vi "Mindsensors NXTMMX Config.vi"(10 "Node Data":T2, 11 "NXT":T3) -> ()   [LabVIEW 2010]
uses:
  <vilib>/NXT/Subs/LVHSConnector.ctl
  Datatypes/Node.ctl
  UI Controls/PlugInControls/Pluginbackground.ctl
  <vilib>/NXT/Block Support/nxt.ctl
  <vilib>/Utility/miscctls.llb/LVPointTypeDef.ctl
  <vilib>/NXT/Block Support/HWPage.SensorMode.ctl
  <vilib>/NXT/Block Support/HWPage.SensorType.ctl
  ConvertNodeAddrSensor.vi
panel:
  out "error out":errorcluster
  out "NXTObject dup":T1 {"nxtIterHandle" format="%08x"; "modIterHandle" format="%08x"; "moduleHandle" format="%08x"; "fileIterHandle" format="%08x"; "fileHandle" format="%08x"; "nxtHandle" format="%08x"}
  in  "Motor Control":string
  in  "Motor 2 Power":i32 min=-100 max=100 step=1
  in  "Motor 1 Power":i32 min=-100 max=100 step=1
  in  "Device Addr":u8=176 format="%x"
  out "Input":dbl format="%#.2g"
  out "number":i8
  in  "Device Address":string
  in  "NXT Port":string
  in  "Name":string
  out "Headline":string="Type (auto populated)"
  in  "Sensor Parameters":string
  in  "Instance Specific Data":cluster{"Example Data":dbl, "Numeric":dbl}
  in  "Reset":bool
  in  "Save":bool
  in  "Stop":bool
  out "Background":T4=TRUE
  # "<- No controls below this line"
  # "Common controls such as Buttons, Rings, Sliders, Graphs, Decorations, etc can be found in the <labview>\\Targets\\NI\\NXT\\NXT Toolkit\\Schematic Editor\\UI Controls\\Plugin Controls\\ folder. Use these controls when possible to ensure a consistent look and feel with LabVIEW Education Edition."
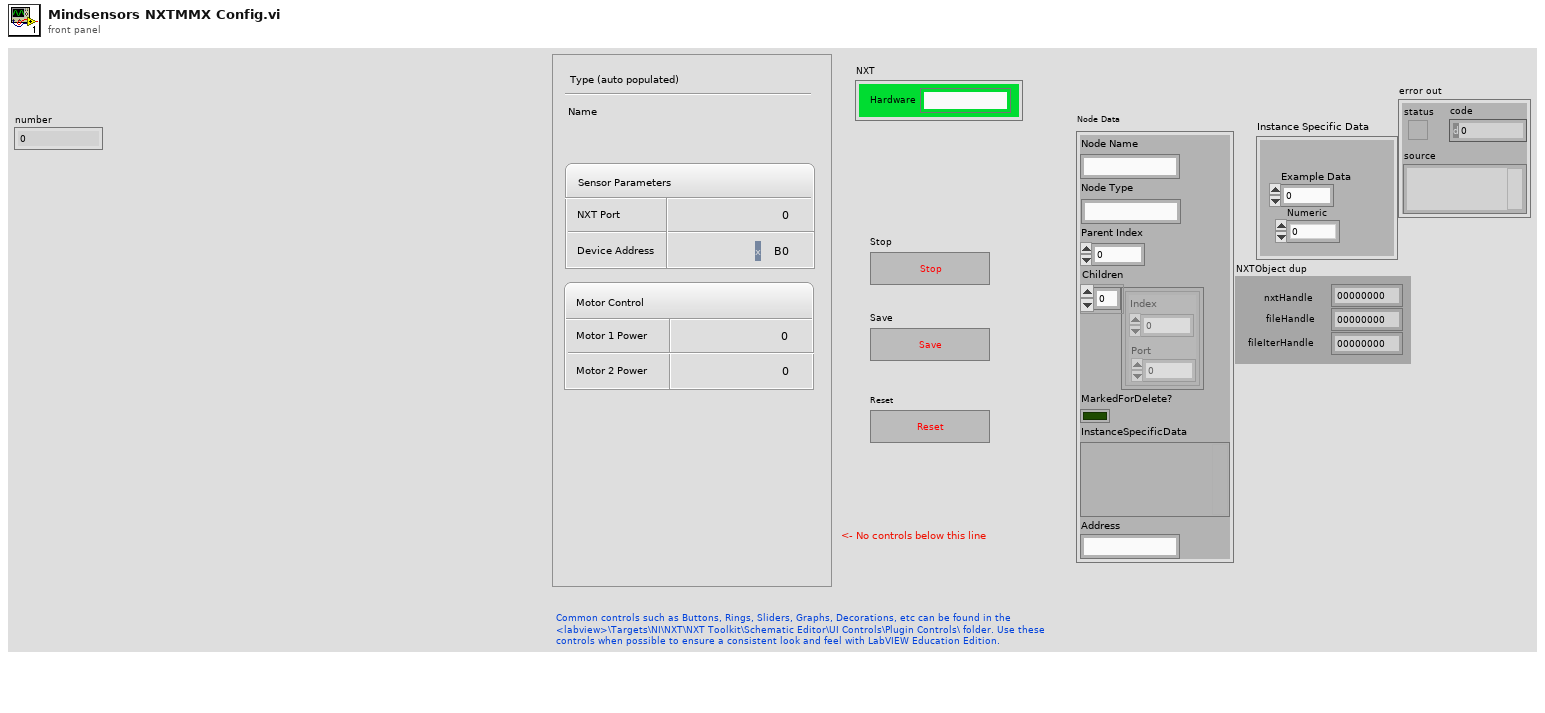
[diagram p1: front panel]
types:
  T1 = typedef "nxt.ctl" = cluster{"nxtHandle":u32, "fileHandle":u32, "fileIterHandle":u32, "moduleHandle":u32, "modIterHandle":u32, "nxtIterHandle":u32}
  T2 = typedef "Node.ctl" = cluster{"Node Name":string, "Node Type":string, "Parent Index":i16, "Children":cluster{"Index":u16, "Port":u16}[], "MarkedForDelete?":bool, "InstanceSpecificData":variant, "Address":string}
  T3 = typedef "LVHSConnector.ctl" = cluster{"Hardware":string, "Flattened String":string}
  T4 = typedef "Pluginbackground.ctl" = bool
  T5 = typedef "LVPointTypeDef.ctl" = cluster{"Horizontal":i16, "Vertical":i16}
  T6 = enum8{"Enabled", "Disabled", "Disabled and Grayed Out"}
  T7 = typedef "HWPage.SensorMode.ctl" = u8
  T8 = typedef "HWPage.SensorType.ctl" = u8
  T9 = typedef "NXT_InputPort.ctl" = u8
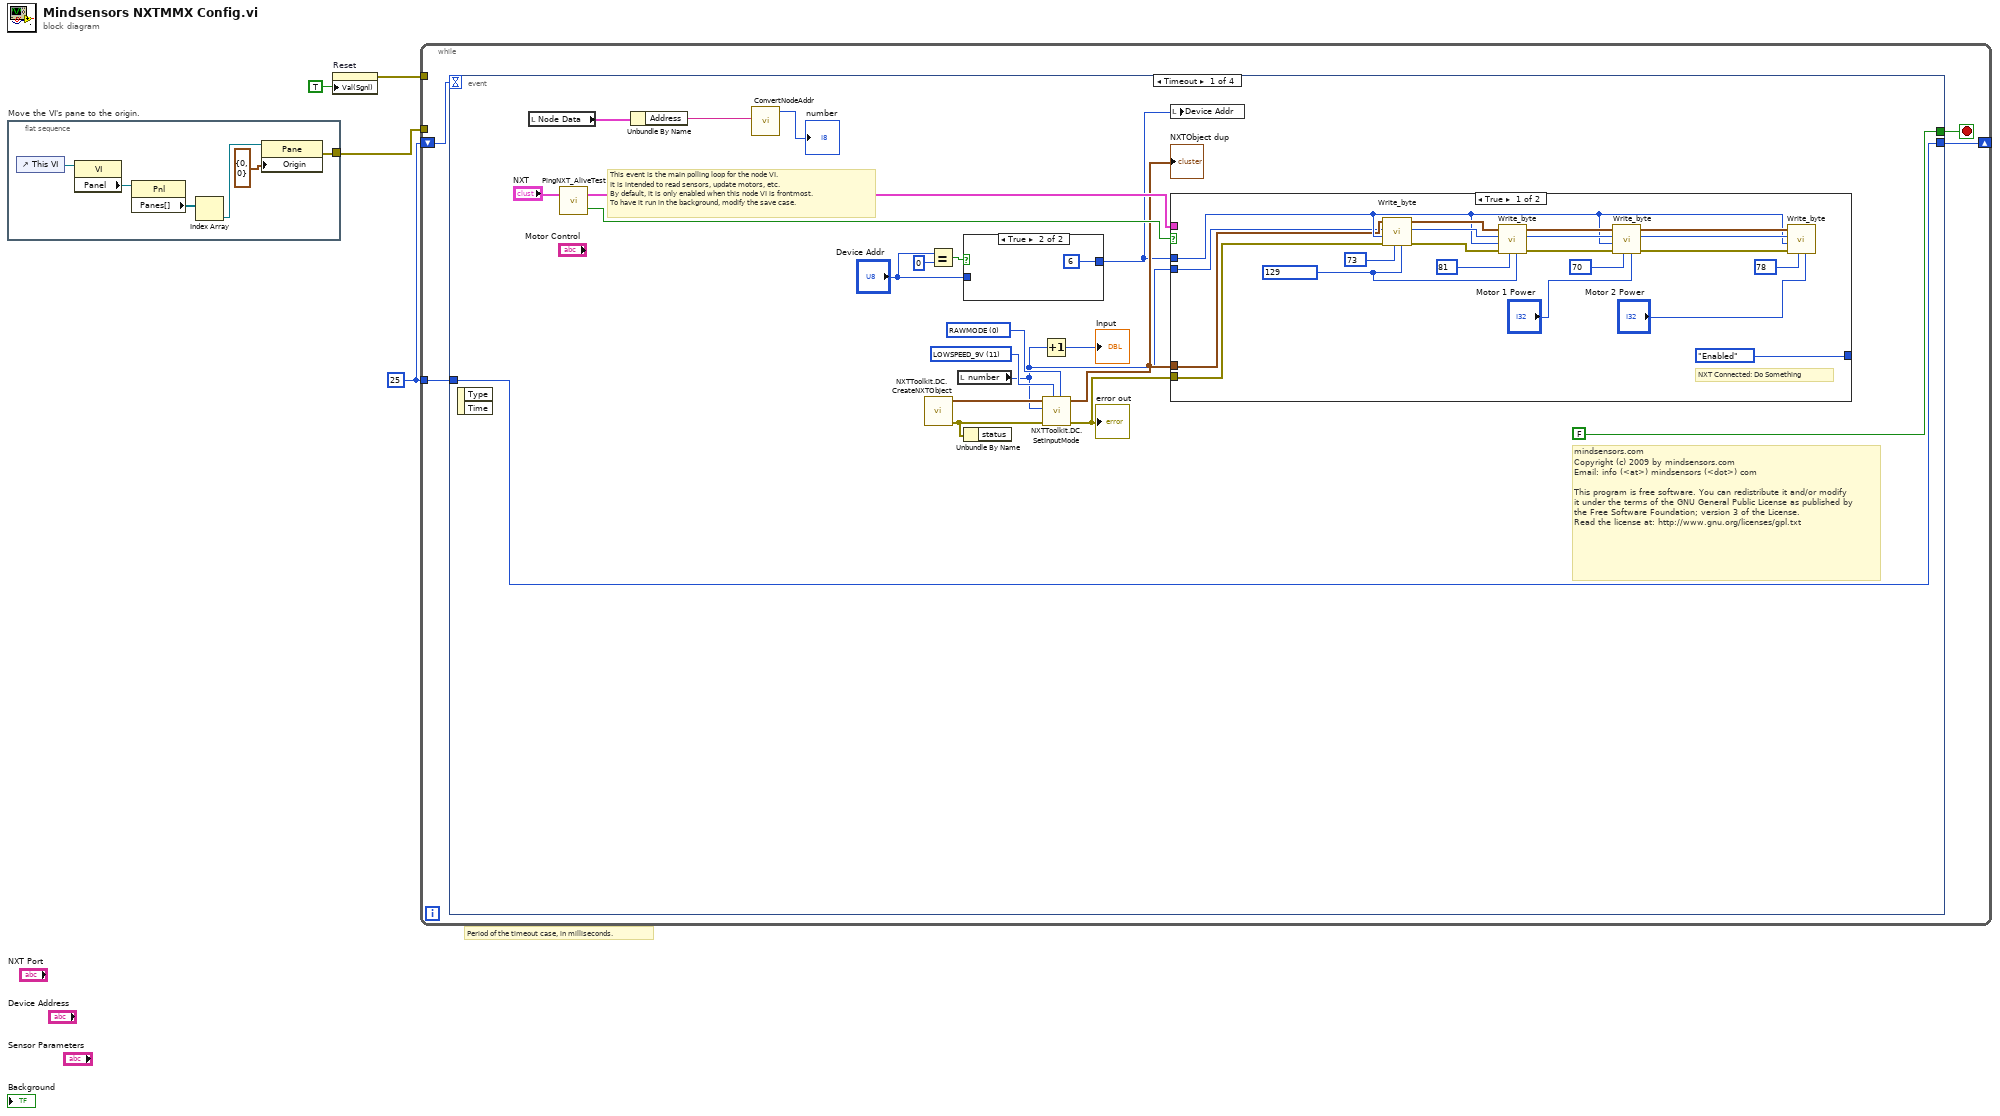
[diagram p0: block diagram]
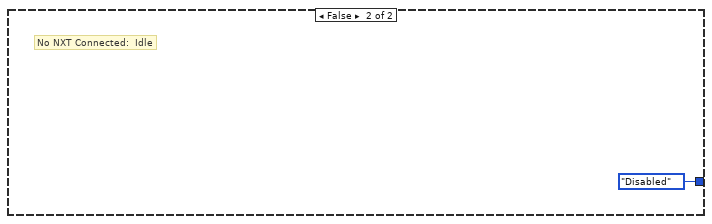
[diagram p3: hidden frame]
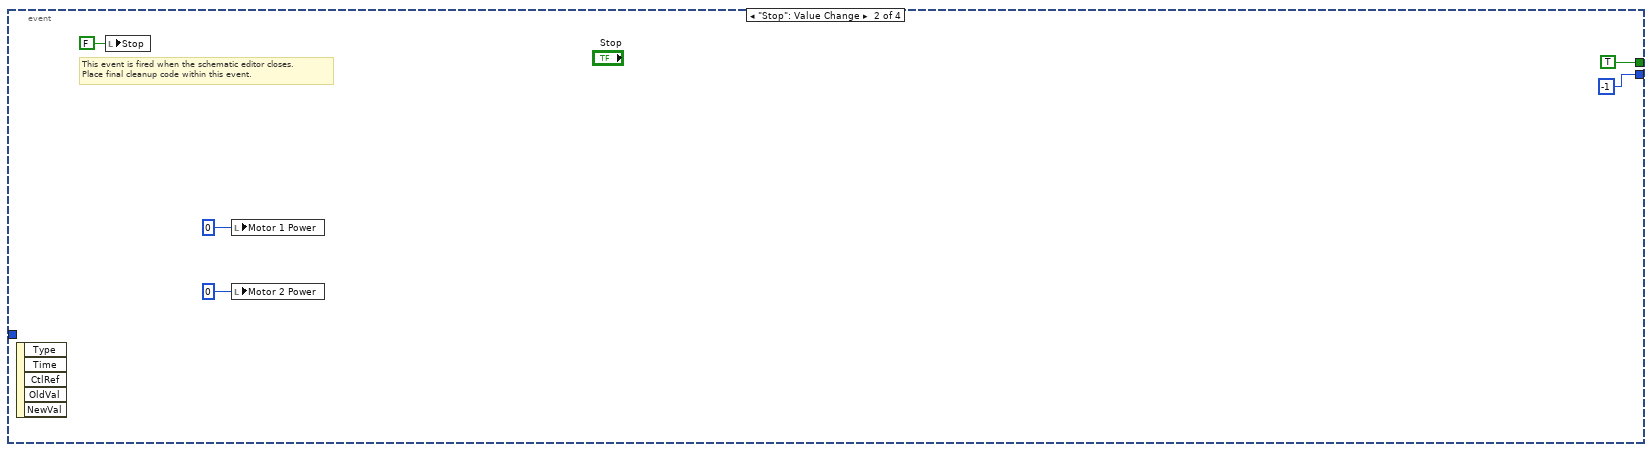
[diagram p4: hidden frame]
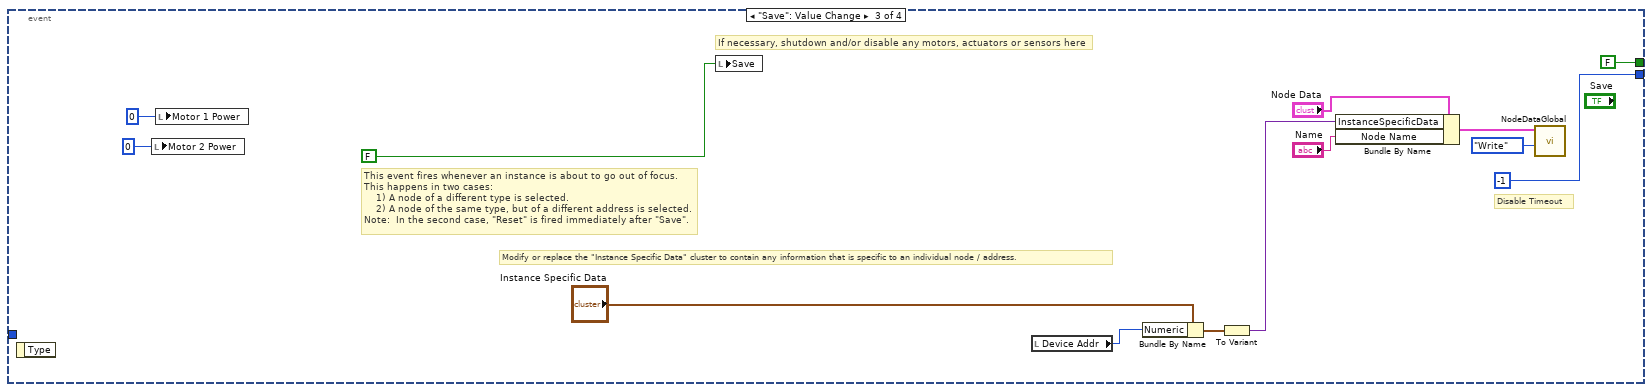
[diagram p5: hidden frame]
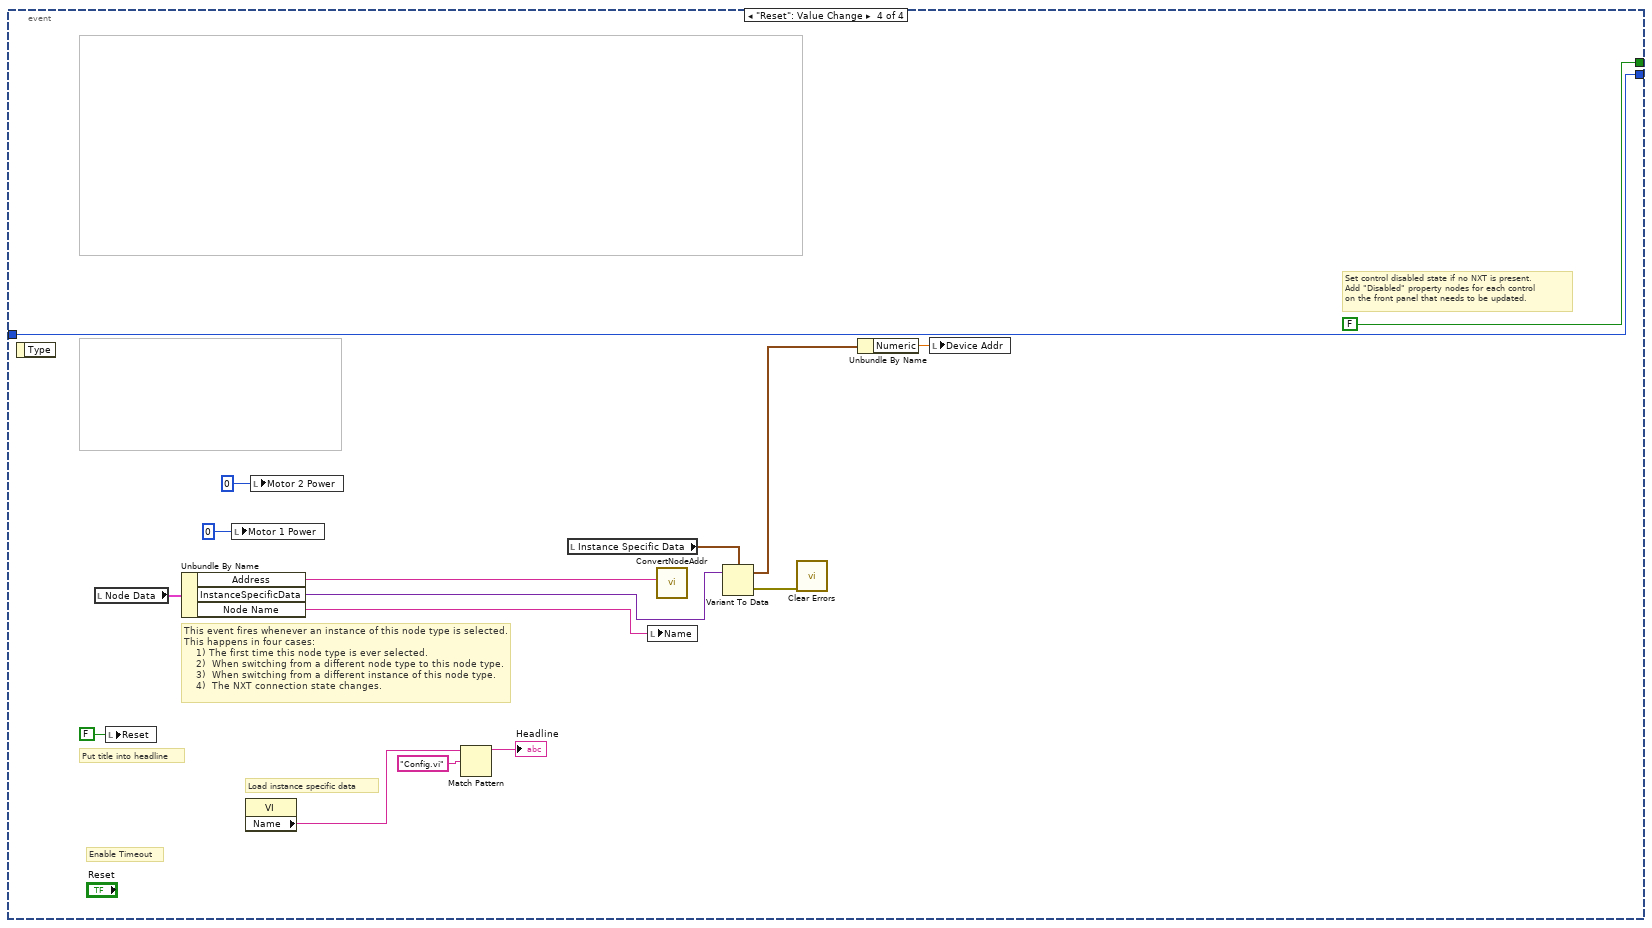
[diagram p6: hidden frame]
diagram:
  w2 = 25
  # "Period of the timeout case, in milliseconds."
  n1 = flat-sequence "Move the VI's pane to the origin." {
    tunnel: [w5] -> w1
    frame #0 {
      n2 = control-ref of="This VI"() -> (w6:refnum<vi>)
      n3 = property class="VI"(reference=w6) -> ("Panel"=w7:refnum<vi>)  [unwired: 1 in, 2 out]
      n4 = property class="Pnl"(reference=w7) -> ("Panes[]"=w8:refnum<vi>[])  [unwired: 1 in, 2 out]
      n5 = Index Array(array=w8) -> (element=w9:refnum<vi>)  [unwired: 1 in]
      n6 = property class="Pane"(reference=w9, "Origin"=T5 {"Horizontal"=0, "Vertical"=0}) -> (error out=w5:errorcluster)  [unwired: 1 in, 1 out]
    }
  }
  n7 = property on="Reset" class="Bool (strict)"("Val(Sgnl)"=TRUE ("Value (Signaling)")) -> (error out=w3:errorcluster)  [unwired: 2 in, 1 out]
  n8 = while {
    tunnel: w3 -> [_]
    shift-right: [w12] -> _
    shift-left: w2 -> [w13]
    tunnel: w2 -> [w11]
    tunnel: w1 -> [_]
    stop <- w14 stop-if-true
    n9 = event shown="[0] Timeout" {
      selector: _ -> [_ _ _ _]
      dyn-events: _ -> [_ _ _ _]
      timeout: w13 -> [_ _ _ _]
      tunnel: [FALSE TRUE FALSE FALSE] -> w14
      tunnel: [w33 -1 -1 w88] -> w12
      tunnel: w11 -> [w33 _ _ w88]
      event Timeout {
        w28 = T7 0 items=["RAWMODE"=0, "BOOLEANMODE"=32, "TRANSITIONCNTMODE"=64, "PERIODCOUNTERMODE"=96, "PCTFULLSCALEMODE"=128, "CELSIUSMODE"=160, "FAHRENHEITMODE"=192, "ANGLESTEPMODE"=224] ("Sensor Mode (RAWMODE)")
        w27 = T8 11 items=["NO_SENSOR", "SWITCH", "TEMPERATURE", "REFLECTION", "ANGLE", "LIGHT_ACTIVE", "LIGHT_INACTIVE", "SOUND_DB", "SOUND_DBA", "CUSTOM", "LOWSPEED", "LOWSPEED_9V", "HIGHSPEED"] ("Sensor Type (NO_SENSOR)")
        # "mindsensors.com\nCopyright (c) 2009 by mindsensors.com\nEmail: info (<at>) mindsensors (<dot>) com\n\nThis program is free software. You can redistribute it and/or modify\nit under the terms of the GNU General Public License as published by\nthe Free Software Foundation; version 3 of the License.\nRead the license at: http://www.gnu.org/licenses/gpl.txt"
        # "This event is the main polling loop for the node VI.\nIt is intended to read sensors, update motors, etc.\nBy default, it is only enabled when this node VI is frontmost.\nTo have it run in the background, modify the save case."
        n10 = event-data() -> ()  [unwired: 1 in, 2 out]
        n11 = local read "Node Data"() -> (w31:T2)
        n12 = call <vilib>:"PingNXT_AliveTest.vi"("NXT"="NXT") -> ("connected?"=w30:bool, "NXT"=w29:T3)  [unwired: 1 in]
        n13 = Unbundle By Name(w31) -> ("Address"=w18:string)
        n14 = call-poly "ConvertNodeAddr.vi"("Sensor Port"=w18) -> ("NXT Port"=→"number":T9)  [unwired: 6 in, 4 out]
        n15 = call <vilib>:"NXTToolkit.DC.CreateNXTObject.vi"() -> ("error out"=w25:errorcluster, "NXTObject"=w26:T1)  [unwired: 9 in, 1 out]
        n16 = Equal?(x="Device Addr", y=u8 0) -> (x = y?=w21:bool)
        n17 = local read "number"() -> (w16:i8)
        n18 = case shown="True" w21 {
          tunnel: [w35 u8 6 ("Device Addr 2")] -> w19
          tunnel: "Device Addr" -> [w35 _]
          frame False {
          }
          frame True {
          }
        }
        n19 = Unbundle By Name(w25) -> ()  [unwired: 1 out]
        n20 = Increment(x=w16) -> (x+1=→"Input":i8)
        n21 = call <vilib>:"NXTToolkit.DC.SetInputMode.vi"("Sensor Mode (RAWMODE)"=w28, "Sensor Type (NO_SENSOR)"=w27, "error in (no error)"=w25, "Input Port (Port 1)"=w16, "NXTObject"=w26) -> ("error out"=w23:errorcluster, "NXTObject dup"=w24:T1)  [unwired: 4 in, 1 out]
        "NXTObject dup" <- w24
        "error out" <- w23
        n22 = local write "Device Addr"(w19) -> ()
        n23 = case shown="True" w30 {
          tunnel: [T6."Enabled" ("Disabled") T6."Disabled" ("Disabled")] -> _
          tunnel: w29 -> [_ _]
          tunnel: w24 -> [w39 _]
          tunnel: w23 -> [w38 _]
          tunnel: w16 -> [w37 _]
          tunnel: w19 -> [w40 _]
          frame True {
            w41 = u8 129 ("Reg Address")
            # "NXT Connected: Do Something"
            n24 = call <vilib>:"Write_byte.vi"("Data byte"=w41, "Reg Address"=u8 73, "error in (no error)"=w38, "Device Address"=w40, "Input Port in"=w37, "NXTObject"=w39) -> ("error out"=w48:errorcluster, "Input Port dup"=w47:T9, "NXTObject dup"=w49:T1)  [unwired: 1 in, 2 out]
            n25 = call <vilib>:"Write_byte.vi"("Data byte"=w41, "Reg Address"=u8 81, "error in (no error)"=w48, "Device Address"=w40, "Input Port in"=w47, "NXTObject"=w49) -> ("error out"=w43:errorcluster, "Input Port dup"=w42:T9, "NXTObject dup"=w44:T1)  [unwired: 1 in, 2 out]
            n26 = call <vilib>:"Write_byte.vi"("Data byte"="Motor 1 Power", "Reg Address"=u8 70, "error in (no error)"=w43, "Device Address"=w40, "Input Port in"=w42, "NXTObject"=w44) -> ("error out"=w53:errorcluster, "Input Port dup"=w52:T9, "NXTObject dup"=w54:T1)  [unwired: 1 in, 2 out]
            n27 = call <vilib>:"Write_byte.vi"("Data byte"="Motor 2 Power", "Reg Address"=u8 78, "error in (no error)"=w53, "Device Address"=w40, "Input Port in"=w52, "NXTObject"=w54) -> ()  [unwired: 1 in, 5 out]
          }
          frame False {
            # "No NXT Connected:  Idle"
          }
        }
      }
      event "Stop": Value Change {
        # "This event is fired when the schematic editor closes.\nPlace final cleanup code within this event."
        n28 = event-data() -> ()  [unwired: 1 in, 5 out]
        n29 = local write "Stop"(FALSE ("stop")) -> ()
        n30 = local write "Motor 1 Power"(0 ("Motor 1 Power")) -> ()
        n31 = local write "Motor 2 Power"(0 ("Motor 2 Power")) -> ()
      }
      event "Save": Value Change {
        # "If necessary, shutdown and/or disable any motors, actuators or sensors here"
        # "Modify or replace the \"Instance Specific Data\" cluster to contain any information that is specific to an individual node / address."
        # "Disable Timeout"
        # "This event fires whenever an instance is about to go out of focus.\nThis happens in two cases:\n    1) A node of a different type is selected.\n    2) A node of the same type, but of a different address is selected.\nNote:  In the second case, \"Reset\" is fired immediately after \"Save\"."
        n32 = event-data() -> ()  [unwired: 1 in, 1 out]
        n33 = local write "Motor 2 Power"(0 ("Motor 2 Power")) -> ()
        n34 = local write "Motor 1 Power"(0 ("Motor 1 Power")) -> ()
        n35 = local write "Save"(FALSE ("stop")) -> ()
        n36 = local read "Device Addr"() -> (w66:u8)
        n37 = Bundle By Name(cluster="Instance Specific Data", "Numeric"=w66) -> (w67:cluster{"Example Data":dbl, "Numeric":dbl})
        n38 = To Variant(anything=w67) -> (Variant=w74:variant)
        n39 = Bundle By Name(cluster="Node Data", "InstanceSpecificData"=w74, "Node Name"="Name") -> (w73:T2)
        n40 = call "NodeDataGlobal.vi"("Action"=enum16{"Read", "Write"}."Write", "Node Data In"=w73) -> ()  [unwired: 8 in, 2 out]
      }
      event "Reset": Value Change {
        # "Set control disabled state if no NXT is present.\nAdd \"Disabled\" property nodes for each control\non the front panel that needs to be updated."
        # "Load instance specific data"
        # "Enable Timeout"
        # "This event fires whenever an instance of this node type is selected.\nThis happens in four cases:\n    1) The first time this node type is ever selected.\n    2)  When switching from a different node type to this node type.\n    3)  When switching from a different instance of this node type. \n    4)  The NXT connection state changes."
        # "Put title into headline"
        n41 = event-data() -> ()  [unwired: 1 in, 1 out]
        n42 = local read "Node Data"() -> (w89:T2)
        n43 = local write "Reset"(FALSE ("Reset")) -> ()
        n44 = Unbundle By Name(w89) -> ("Address"=w80:string, "InstanceSpecificData"=w90:variant, "Node Name"=w82:string)
        n45 = local write "Motor 1 Power"(0 ("Motor 1 Power")) -> ()
        n46 = property class="VI"() -> ("Name"=w84:string)  [unwired: 2 in, 2 out]
        n47 = local write "Motor 2 Power"(0 ("Motor 2 Power")) -> ()
        n48 = Match Pattern(string=w84, regular expression="Config.vi") -> (before substring=→"Headline":string)  [unwired: 1 in, 3 out]
        n49 = local read "Instance Specific Data"() -> (w87:cluster{"Example Data":dbl, "Numeric":dbl})
        n50 = local write "Name"(w82) -> ()
        n51 = call-poly "ConvertNodeAddr.vi"("Sensor Port"=w80) -> ()  [unwired: 6 in, 5 out]
        n52 = Variant To Data(Variant=w90, type=w87) -> (error out=w86:errorcluster, data=w81:cluster{"Example Data":dbl, "Numeric":dbl})  [unwired: 1 in]
        n53 = call <vilib>:"Clear Errors.vi"("error in (no error)"=w86) -> ()  [unwired: 6 in, 1 out]
        n54 = Unbundle By Name(w81) -> ("Numeric"=w79:dbl)
        n55 = local write "Device Addr"(w79) -> ()
      }
    }
  }
